vi "week03_Ex02.vi"() -> ()   [LabVIEW 2017]
panel:
  out "all lower case string":string
  out "substring":string
  out "length 2":i32
  out "String Out 1":string
  out "length":i32
  in  "String  1":string
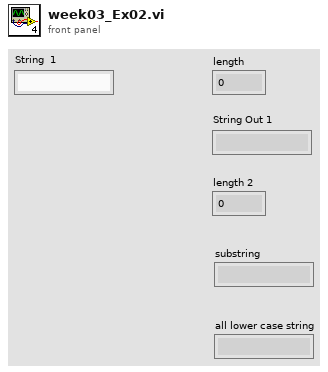
[diagram p1: front panel]
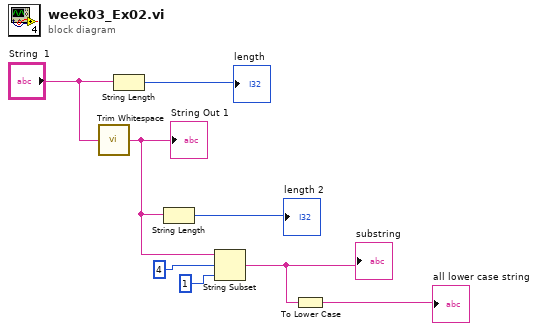
[diagram p0: block diagram]
diagram:
  n1 = call <vilib>:"Trim Whitespace.vi"("string"="String  1") -> ("trimmed string"=w5:string)  [unwired: 1 in]
  "String Out 1" <- w5
  n2 = String Length(string="String  1") -> (length=→"length":i32)
  n3 = String Length(string=w5) -> (length=→"length 2":i32)
  n4 = String Subset(string=w5, offset (0)=4, length (rest)=1 ("length (rest)")) -> (substring=w2:string)
  "substring" <- w2
  n5 = To Lower Case(string=w2) -> (all lower case string=→"all lower case string":string)
